vi "Automatic Teller Machine (ATM).vi"() -> ()   [LabVIEW 2019]
uses:
  Controls/UI Data.ctl
  Controls/Message selector.ctl
  SubVIs/FGV Selector.ctl
  SubVIs/Operation.ctl
  Controls/Write Menu.ctl
  support/Message Queue/Enqueue Message (Single).vi
  <vilib>/Utility/file.llb/Read Delimited Spreadsheet (string).vi
  <vilib>/Utility/file.llb/Write Delimited Spreadsheet (string).vi
  <vilib>/Utility/error.llb/Error Cluster From Error Code.vi
  <vilib>/ErrorRing/Error Ring.xnode
  support/Message Queue/Message Queue.lvlib
  support/User Event - Stop/User Event - Stop.lvlib
panel:
  in  "Enter":bool
  in  "User Input":string
  in  "Right Buttons":T1
  out "Right Menu":T2
  in  "Left Buttons":T1
  out "Left Menu":T2
  in  "Card Simulator":bool
  out "ATM Messages":string
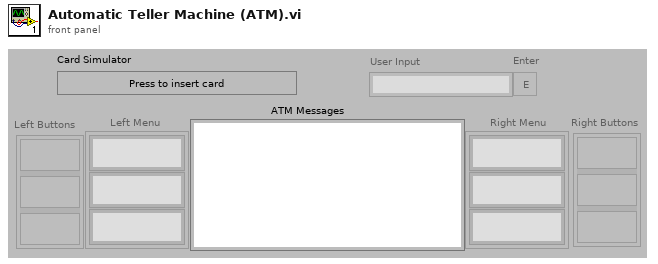
[diagram p1: front panel]
types:
  T1 = cluster{"Func Button":bool, "Func Button 2":bool, "Func Button 3":bool}
  T2 = cluster{"RFS String":string, "RFS String 2":string, "RFS String 3":string}
  T3 = typedef "UI Data.ctl" = cluster{"Account":string, "First Name":string, "Last Name":string, "Cash":i32}
  T4 = typedef "Message Queue.lvlib/All Message Queues.ctl" = cluster{"UI":refnum<queue>}
  T5 = typedef "Operation.ctl" = enum16{"No item", "Card Inserted", "Deposit", "Withdrawn"}
  T6 = typedef "FGV Selector.ctl" = enum16{"Set", "Get"}
  T7 = typedef "Message selector.ctl" = enum16{"Welcome Message", "Main Menu Message", "Account Verification Failed Message", "Session Terminate Message", "Deposit Message", "Deposit Complete Message", "Withdrawal Message", "Withdrawal Complete Message", "Withdrawal Failed Message", "Balance Inquiry Message"}
  T8 = typedef "Write Menu.ctl" = enum16{"Empty Value", "Standard Value"}
  T9 = enum8{"Enabled", "Disabled", "Disabled and Grayed Out"}
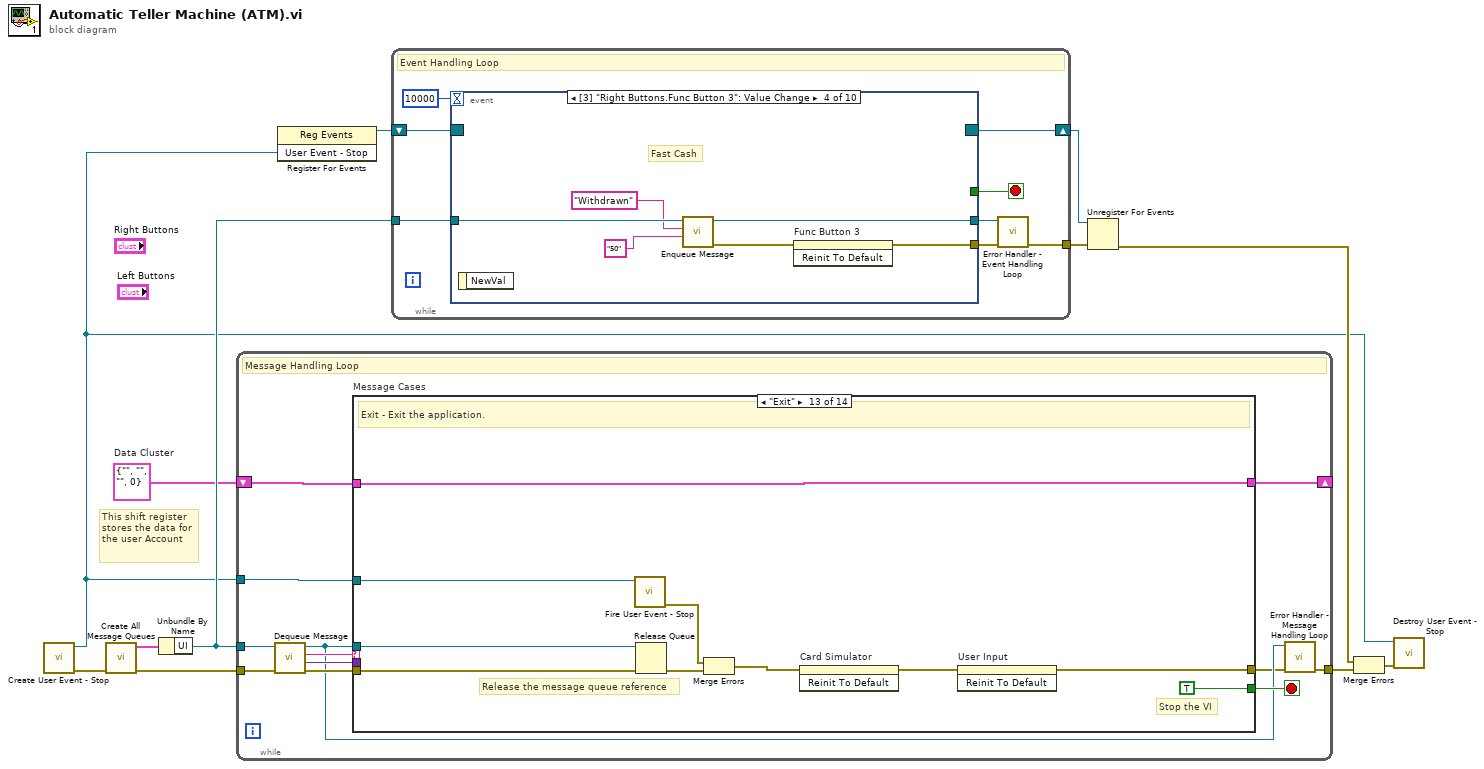
[diagram p0: block diagram]
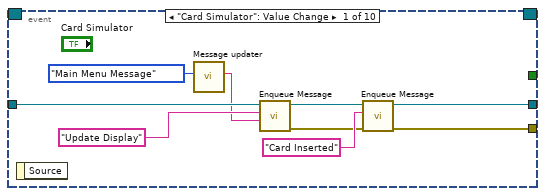
[diagram p2: hidden frame]
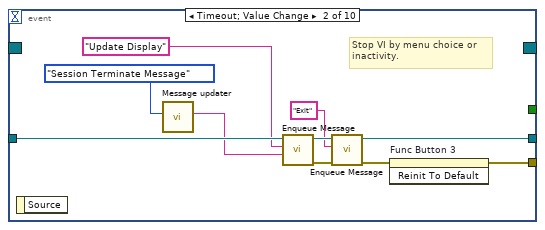
[diagram p3: hidden frame]
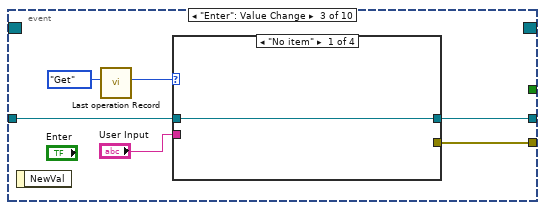
[diagram p4: hidden frame]
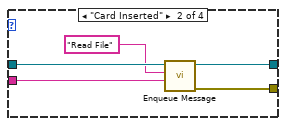
[diagram p5: hidden frame]
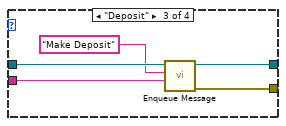
[diagram p6: hidden frame]
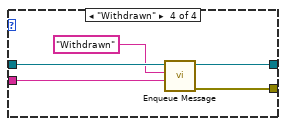
[diagram p7: hidden frame]
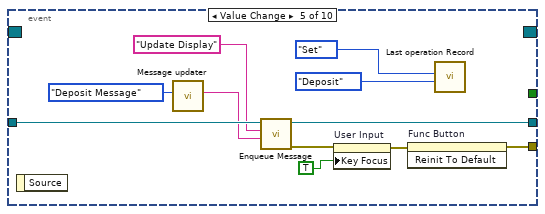
[diagram p8: hidden frame]
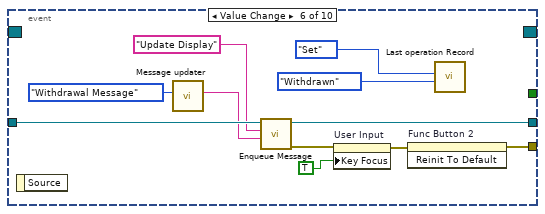
[diagram p9: hidden frame]
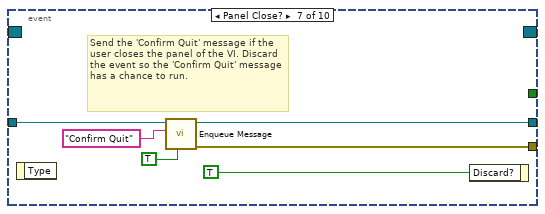
[diagram p10: hidden frame]
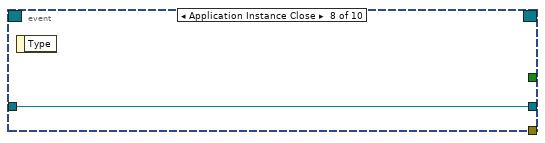
[diagram p11: hidden frame]
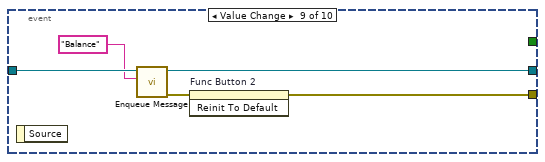
[diagram p12: hidden frame]
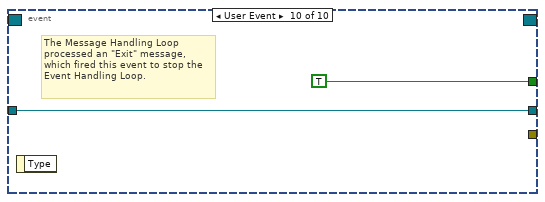
[diagram p13: hidden frame]
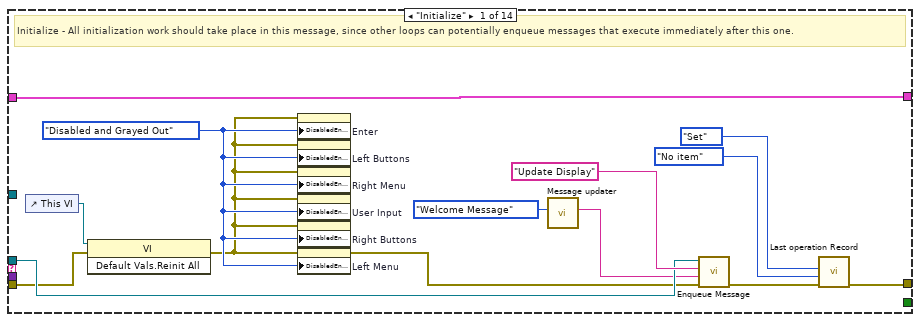
[diagram p14: hidden frame]
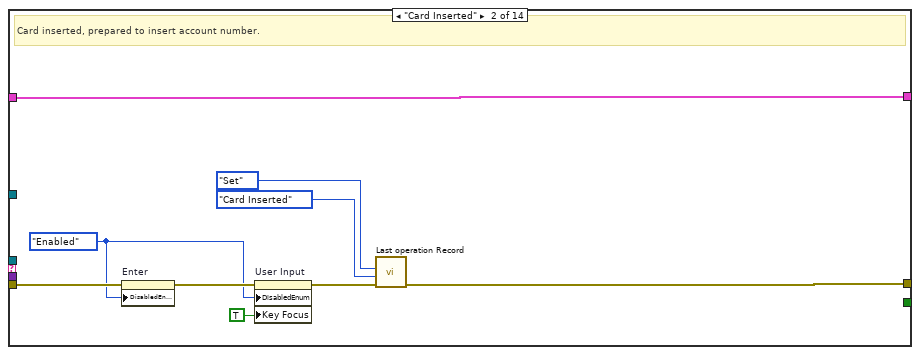
[diagram p15: hidden frame]
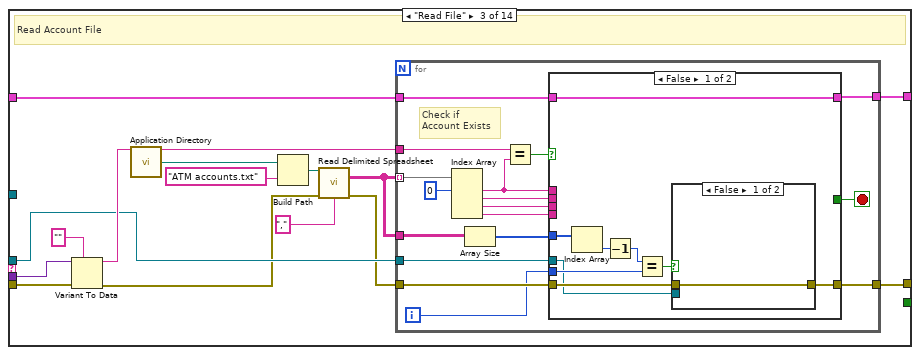
[diagram p16: hidden frame]
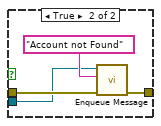
[diagram p17: hidden frame]
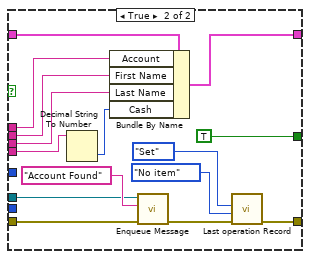
[diagram p18: hidden frame]
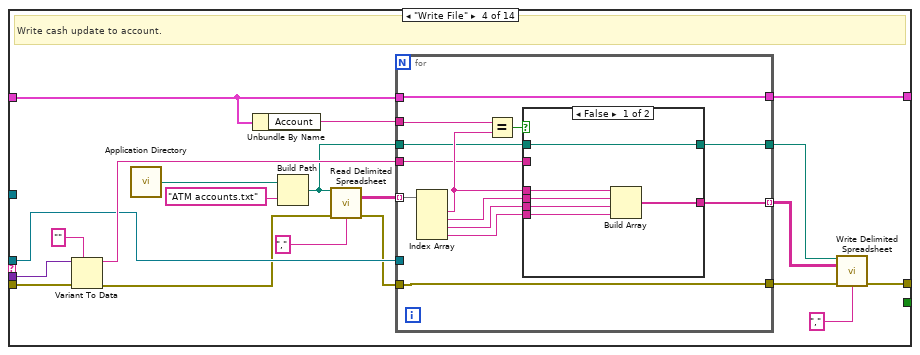
[diagram p19: hidden frame]
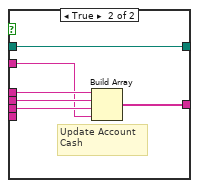
[diagram p20: hidden frame]
diagram:
  w4 = T3 {"Account"="", "First Name"="", "Last Name"="", "Cash"=0}  # Data Cluster
  # "This shift register stores the data for the user Account"
  n1 = call "Create User Event - Stop.vi"() -> ("error out"=w8:errorcluster, "User Event - Stop"=w1:refnum<user-event>)  [unwired: 10 in]
  n2 = call "Create All Message Queues.vi"("error in (no error)"=w8) -> ("error out"=w12:errorcluster, "Message Queues out"=w11:T4)  [unwired: 9 in]
  n3 = Unbundle By Name(w11) -> ("UI"=w9:refnum<queue>)
  n4 = while {
    tunnel: w9 -> [w16]
    shift-right: [w23] -> _
    shift-left: w4 -> [w24]
    tunnel: w1 -> [w21]
    tunnel: w12 -> [w20]
    tunnel: [w14] -> w10
    stop <- w22 stop-if-true
    # "Message Handling Loop"
    n5 = call "Dequeue Message.vi"("error in (no error)"=w20, "Message Queue"=w16) -> ("error out"=w19:errorcluster, "Message Data"=w17:variant, "Message"=w18:string, "dup Message Queue"=w15:refnum<queue>)  [unwired: 6 in]
    n6 = case "Message Cases" shown="\"Exit\"" w18 {
      selector: w18 -> [_ _ _ _ _ _ _ _ _ _ _ _ _ w292]
      tunnel: w15 -> [w36 _ w51 w121 w170 w183 w193 w220 w237 _ _ w278 w291 _]
      tunnel: w19 -> [w31 w45 w58 w125 w166 w181 w190 w215 w236 w268 w275 w281 w285 _]
      tunnel: [w27 w42 w53 w111 w179 w186 w197 w205 w230 w263 w270 w279 w282 w293] -> w13
      tunnel: w24 -> [w38 w47 w54 w117 w175 w184 w195 w209 w232 w269 w274 w280 w290 w294]
      tunnel: [w38 w47 w52 w114 w175 w184 w195 w207 w231 w269 w274 w280 w290 w294] -> w23
      tunnel: [_ _ _ _ _ _ _ _ _ _ _ _ TRUE _] -> w22
      tunnel: w17 -> [_ _ w57 w124 _ _ _ w214 w235 w267 w273 _ _ _]
      tunnel: w21 -> [_ _ _ _ _ _ _ _ _ _ _ _ w287 _]
      frame "Initialize" {
        w33 = T9."Disabled and Grayed Out" ("Disabled")
        # "Initialize - All initialization work should take place in this message, since other loops can potentially enqueue messages that execute immediately after this one."
        n7 = control-ref of="This VI"() -> (w32:refnum<vi>)
        n8 = invoke class="VI" method="Default Vals.Reinit All"(reference=w32, error in=w31) -> (error out=w30:errorcluster)  [unwired: 1 in, 2 out]
        n9 = property on="Enter" class="Bool"(error in=w30, "DisabledEnum"=w33) -> ()  [unwired: 1 in, 2 out]
        n10 = property on="Left Buttons" class="Clust"(error in=w30, "DisabledEnum"=w33) -> ()  [unwired: 1 in, 2 out]
        n11 = property on="Right Menu" class="Clust (strict)"(error in=w30, "DisabledEnum"=w33) -> ()  [unwired: 1 in, 2 out]
        n12 = property on="User Input" class="Str"(error in=w30, "DisabledEnum"=w33) -> ()  [unwired: 1 in, 2 out]
        n13 = property on="Right Buttons" class="Clust"(error in=w30, "DisabledEnum"=w33) -> ()  [unwired: 1 in, 2 out]
        n14 = property on="Left Menu" class="Clust (strict)"(error in=w30, "DisabledEnum"=w33) -> (error out=w29:errorcluster)  [unwired: 1 in, 1 out]
        n15 = call "Message updater.vi"("Message Selector"=Message_selector."Welcome Message") -> ("Message"=w34:string)  [unwired: 10 in]
        n16 = call-poly "Enqueue Message.vi"("error in (no error)"=w29, "Message Data"=w34, "Message"="Update Display", "Message Queue"=w36) -> ("error out"=w28:errorcluster)  [unwired: 6 in, 1 out]
        n17 = call "Last operation Record.vi"("Error In"=w28, "Operation"=Operation."No item", "FGV Choice"=FGV_Selector."Set") -> ("Error Out"=w27:errorcluster)  [unwired: 7 in, 1 out]
      }
      frame "Card Inserted" {
        w44 = T9."Enabled" ("Disabled")
        # "Card inserted, prepared to insert account number."
        n18 = property on="Enter" class="Bool"(error in=w45, "DisabledEnum"=w44) -> (error out=w46:errorcluster)  [unwired: 1 in, 1 out]
        n19 = property on="User Input" class="Str"(error in=w46, "DisabledEnum"=w44, "Key Focus"=TRUE) -> (error out=w43:errorcluster)  [unwired: 1 in, 1 out]
        n20 = call "Last operation Record.vi"("Error In"=w43, "Operation"=Operation."Card Inserted", "FGV Choice"=FGV_Selector."Set") -> ("Error Out"=w42:errorcluster)  [unwired: 7 in, 1 out]
      }
      frame "Read File" {
        # "Read Account File"
        n21 = Variant To Data(error in=w58, type="", Variant=w57) -> (data=w55:string, error out=w50:errorcluster)
        n22 = call <vilib>:"Application Directory.vi"() -> ("Application Directory"=w61:path)
        n23 = Build Path(base path=w61, name or relative path="ATM accounts.txt") -> (appended path=w59:path)
        n24 = call-poly <vilib>:"Read Delimited Spreadsheet.vi"("file path (dialog if empty)"=w59, "error in (no error)"=w50, "delimiter (\\t)"="," ("delimiter (\\t)")) -> ("all rows"=w48:string[][], "error out"=w49:errorcluster)  [unwired: 7 in, 4 out]
        n25 = for {
          tunnel: w48 -> [w79] mode=indexing
          tunnel: w49 -> [w68]
          tunnel: w55 -> [w77]
          tunnel: w54 -> [w75]
          tunnel: [w72] -> w52
          tunnel: [w70] -> w53
          tunnel: w51 -> [w69]
          tunnel: w48 -> [w67]
          i -> [w63]
          stop <- w71 stop-if-true
          # "Check if\nAccount Exists"
          n26 = Index Array(array=w79, index #1=0 ("index")) -> (element #1=w73:string, element #2=w74:string, element #3=w64:string, element #4=w65:string)  [unwired: 3 in]
          n27 = Array Size(array=w67) -> (size(s)=w66:i32[])
          n28 = Equal?(x=w77, y=w73) -> (x = y?=w76:bool)
          n29 = case shown="False" w76 {
            tunnel: w75 -> [w88 w108]
            tunnel: w74 -> [_ w106]
            tunnel: w65 -> [_ w107]
            tunnel: w73 -> [_ w105]
            tunnel: [w88 w104] -> w72
            tunnel: [_ TRUE] -> w71
            tunnel: [w80 w96] -> w70
            tunnel: w69 -> [w81 w101]
            tunnel: w68 -> [w82 w100]
            tunnel: w66 -> [w86 _]
            tunnel: w64 -> [_ w94]
            tunnel: w63 -> [w83 _]
            frame False {
              n30 = Index Array(array=w86) -> (element=w87:i32)  [unwired: 1 in]
              n31 = Decrement(x=w87) -> (x-1=w84:i32)
              n32 = Equal?(x=w84, y=w83) -> (x = y?=w85:bool)
              n33 = case shown="False" w85 {
                tunnel: w82 -> [w89 w92]
                tunnel: w81 -> [_ w91]
                tunnel: [w89 w90] -> w80
                frame False {
                }
                frame True {
                  n34 = call-poly "Enqueue Message.vi"("error in (no error)"=w92, "Message"="Account not Found", "Message Queue"=w91) -> ("error out"=w90:errorcluster)  [unwired: 7 in, 1 out]
                }
              }
            }
            frame True {
              n35 = Decimal String To Number(string=w107) -> (number=w95:i32)  [unwired: 2 in, 1 out]
              n36 = Bundle By Name(cluster=w108, "Account"=w105, "First Name"=w106, "Last Name"=w94, "Cash"=w95) -> (w104:T3)
              n37 = call-poly "Enqueue Message.vi"("error in (no error)"=w100, "Message"="Account Found", "Message Queue"=w101) -> ("error out"=w97:errorcluster)  [unwired: 7 in, 1 out]
              n38 = call "Last operation Record.vi"("Error In"=w97, "Operation"=Operation."No item", "FGV Choice"=FGV_Selector."Set") -> ("Error Out"=w96:errorcluster)  [unwired: 7 in, 1 out]
            }
          }
        }
      }
      frame "Write File" {
        # "Write cash update to account."
        n39 = Variant To Data(error in=w125, type="", Variant=w124) -> (data=w122:string, error out=w120:errorcluster)
        n40 = call <vilib>:"Application Directory.vi"() -> ("Application Directory"=w127:path)
        n41 = Unbundle By Name(w117) -> ("Account"=w116:string)
        n42 = Build Path(base path=w127, name or relative path="ATM accounts.txt") -> (appended path=w115:path)
        n43 = call-poly <vilib>:"Read Delimited Spreadsheet.vi"("file path (dialog if empty)"=w115, "error in (no error)"=w120, "delimiter (\\t)"="," ("delimiter (\\t)")) -> ("all rows"=w118:string[][], "error out"=w119:errorcluster)  [unwired: 7 in, 4 out]
        n44 = for {
          tunnel: w118 -> [w141] mode=indexing
          tunnel: w119 -> [w129]
          tunnel: w122 -> [w133]
          tunnel: w117 -> [w132]
          tunnel: w121 -> [_]
          tunnel: w116 -> [w140]
          tunnel: [w134] -> w112 mode=indexing
          tunnel: w115 -> [w131]
          tunnel: [w132] -> w114
          tunnel: [w130] -> w113
          tunnel: [w129] -> w110
          n45 = Index Array(array=w141) -> (element #1=w138:string, element #2=w137:string, element #3=w136:string, element #4=w135:string)  [unwired: 4 in]
          n46 = Equal?(x=w140, y=w138) -> (x = y?=w139:bool)
          n47 = case shown="False" w139 {
            tunnel: w138 -> [w147 w153]
            tunnel: w137 -> [w146 w152]
            tunnel: w136 -> [w145 w151]
            tunnel: w135 -> [w144 _]
            tunnel: [w143 w150] -> w134
            tunnel: w133 -> [_ w149]
            tunnel: w131 -> [w142 w148]
            tunnel: [w142 w148] -> w130
            frame False {
              n48 = Build Array(w147, w146, w145, w144) -> (w143:string[])
            }
            frame True {
              # "Update Account\nCash"
              n49 = Build Array(w153, w152, w151, w149) -> (w150:string[])
            }
          }
        }
        n50 = call-poly <vilib>:"Write Delimited Spreadsheet.vi"("file path (dialog if empty)"=w113, "2D data"=w112, "error in (no error)"=w110, "delimiter (\\t)"="," ("delimiter (\\t)")) -> ("error out"=w111:errorcluster)  [unwired: 10 in, 1 out]
      }
      frame "Account Found" {
        w167 = T9."Enabled" ("Disabled")
        # "If account was found, enable controls, menus and show message displaying customer name."
        n51 = property on="Left Buttons" class="Clust"(error in=w166, "DisabledEnum"=w167) -> (error out=w163:errorcluster)  [unwired: 1 in, 1 out]
        n52 = property on="Right Menu" class="Clust (strict)"(error in=w166, "DisabledEnum"=w167) -> (error out=w162:errorcluster)  [unwired: 1 in, 1 out]
        n53 = property on="Right Buttons" class="Clust"(error in=w166, "DisabledEnum"=w167) -> (error out=w161:errorcluster)  [unwired: 1 in, 1 out]
        n54 = property on="Left Menu" class="Clust (strict)"(error in=w166, "DisabledEnum"=w167) -> (error out=w160:errorcluster)  [unwired: 1 in, 1 out]
        n55 = Merge Errors(w163, w162, w161, w160) -> (w164:errorcluster)
        n56 = call "Write Menu Value.vi"("Error In"=w164, "Menu Write choice"=Write_Menu."Standard Value") -> ("Error Out"=w157:errorcluster, "Right Menu"=→"Right Menu":T2, "Left Menu"=→"Left Menu":T2)  [unwired: 7 in]
        n57 = call "Last operation Record.vi"("Error In"=w157, "Operation"=Operation."No item", "FGV Choice"=FGV_Selector."Set") -> ("Error Out"=w156:errorcluster)  [unwired: 7 in, 1 out]
        n58 = Unbundle By Name(w175) -> ("Last Name"=w171:string, "First Name"=w173:string)
        n59 = call "Message updater.vi"("Message Selector"=Message_selector."Main Menu Message") -> ("Message"=w177:string)  [unwired: 10 in]
        n60 = Search and Replace String(input string=w177, search string="First Name", replace string=w173) -> (result string=w176:string)  [unwired: 5 in, 3 out]
        n61 = Search and Replace String(input string=w176, search string="Last Name (from file)", replace string=w171) -> (result string=w168:string)  [unwired: 5 in, 3 out]
        n62 = call-poly "Enqueue Message.vi"("error in (no error)"=w156, "Message Data"=w168, "Message"="Update Display", "Message Queue"=w170) -> ("error out"=w179:errorcluster)  [unwired: 6 in, 1 out]
      }
      frame "Account not Found" {
        # "Send message to Display showing that account does not exist."
        n63 = call "Message updater.vi"("Message Selector"=Message_selector."Account Verification Failed Message") -> ("Message"=w180:string)  [unwired: 10 in]
        n64 = call-poly "Enqueue Message.vi"("error in (no error)"=w181, "Message Data"=w180, "Message"="Update Display", "Message Queue"=w183) -> ("error out"=w186:errorcluster)  [unwired: 6 in, 1 out]
      }
      frame "Balance" {
        # "Get Balance From account."
        n65 = Unbundle By Name(w195) -> ("Cash"=w188:i32)
        n66 = call "Message updater.vi"("Message Selector"=Message_selector."Balance Inquiry Message") -> ("Message"=w189:string)  [unwired: 10 in]
        n67 = Number To Decimal String(number=w188) -> (decimal integer string=w187:string)  [unwired: 1 in]
        n68 = Search and Replace String(input string=w189, search string="(Balance Amount from file)", replace string=w187) -> (result string=w191:string)  [unwired: 5 in, 3 out]
        n69 = call-poly "Enqueue Message.vi"("error in (no error)"=w190, "Message Data"=w191, "Message"="Update Display", "Message Queue"=w193) -> ("error out"=w197:errorcluster)  [unwired: 6 in, 1 out]
      }
      frame "Make Deposit" {
        # "Make Deposit"
        n70 = Unbundle By Name(w209) -> ("Cash"=w211:i32)
        n71 = Variant To Data(error in=w215, type="", Variant=w214) -> (data=w212:string, error out=w199:errorcluster)
        n72 = Decimal String To Number(string=w212) -> (number=w210:i32)  [unwired: 2 in, 1 out]
        n73 = Add(x=w211, y=w210) -> (x+y=w208:i32)
        n74 = Bundle By Name(cluster=w209, "Cash"=w208) -> (w207:T3)
        n75 = call "Last operation Record.vi"("Error In"=w199, "Operation"=Operation."No item", "FGV Choice"=FGV_Selector."Set") -> ("Error Out"=w198:errorcluster)  [unwired: 7 in, 1 out]
        n76 = Unbundle By Name(w207) -> ("Cash"=w216:i32)
        n77 = Number To Decimal String(number=w216) -> (decimal integer string=w202:string)  [unwired: 1 in]
        n78 = call "Message updater.vi"("Message Selector"=Message_selector."Deposit Complete Message") -> ("Message"=w217:string)  [unwired: 10 in]
        n79 = Search and Replace String(input string=w217, search string="(Amount)", replace string=w212) -> (result string=w218:string)  [unwired: 5 in, 3 out]
        n80 = call-poly "Enqueue Message.vi"("error in (no error)"=w198, "Message Data"=w218, "Message"="Update Display", "Message Queue"=w220) -> ("error out"=w204:errorcluster, "dup Message Queue"=w206:refnum<queue>)  [unwired: 6 in]
        n81 = call-poly "Enqueue Message.vi"("error in (no error)"=w204, "Message Data"=w202, "Message"="Write File", "Message Queue"=w206) -> ("error out"=w205:errorcluster)  [unwired: 6 in, 1 out]
      }
      frame "Withdrawn" {
        # "Make Deposit"
        n82 = Variant To Data(error in=w236, type="", Variant=w235) -> (data=w233:string, error out=w224:errorcluster)
        n83 = Unbundle By Name(w232) -> ("Cash"=w228:i32)
        n84 = Decimal String To Number(string=w233) -> (number=w227:i32)  [unwired: 2 in, 1 out]
        n85 = Greater Or Equal?(x=w228, y=w227) -> (x >= y?=w229:bool)
        n86 = call "Last operation Record.vi"("Error In"=w224, "Operation"=Operation."No item", "FGV Choice"=FGV_Selector."Set") -> ("Error Out"=w223:errorcluster)  [unwired: 7 in, 1 out]
        n87 = case shown="True" w229 {
          tunnel: w237 -> [w253 w261]
          tunnel: w223 -> [w249 w258]
          tunnel: w233 -> [w248 _]
          tunnel: w232 -> [w247 w257]
          tunnel: [w246 w257] -> w231
          tunnel: [w244 w256] -> w230
          tunnel: w228 -> [w240 _]
          tunnel: w227 -> [w239 _]
          frame True {
            n88 = Subtract(x=w240, y=w239) -> (x-y=w238:i32)
            n89 = Bundle By Name(cluster=w247, "Cash"=w238) -> (w246:T3)
            n90 = Number To Decimal String(number=w238) -> (decimal integer string=w241:string)  [unwired: 1 in]
            n91 = call "Message updater.vi"("Message Selector"=Message_selector."Withdrawal Complete Message") -> ("Message"=w250:string)  [unwired: 10 in]
            n92 = Search and Replace String(input string=w250, search string="(Amount)", replace string=w248) -> (result string=w251:string)  [unwired: 5 in, 3 out]
            n93 = call-poly "Enqueue Message.vi"("error in (no error)"=w249, "Message Data"=w251, "Message"="Update Display", "Message Queue"=w253) -> ("error out"=w243:errorcluster, "dup Message Queue"=w245:refnum<queue>)  [unwired: 6 in]
            n94 = call-poly "Enqueue Message.vi"("error in (no error)"=w243, "Message Data"=w241, "Message"="Write File", "Message Queue"=w245) -> ("error out"=w244:errorcluster)  [unwired: 6 in, 1 out]
          }
          frame False {
            n95 = call "Message updater.vi"("Message Selector"=Message_selector."Withdrawal Failed Message") -> ("Message"=w259:string)  [unwired: 10 in]
            n96 = call-poly "Enqueue Message.vi"("error in (no error)"=w258, "Message Data"=w259, "Message"="Update Display", "Message Queue"=w261) -> ("error out"=w256:errorcluster)  [unwired: 6 in, 1 out]
          }
        }
      }
      frame "Update Display" {
        # "Update Display - Convert the message data to a string to display in the Data Display indicator."
        n97 = Variant To Data(error in=w268, type="", Variant=w267) -> (data=→"ATM Messages":string, error out=w264:errorcluster)
        n98 = invoke on="User Input" class="Str" method="Reinit To Default"(error in=w264) -> (error out=w263:errorcluster)  [unwired: 2 in, 2 out]
      }
      frame "Error" {
        # "Error - Display an error dialog. This message is sent by the \"Error Handler\" VIs at the end of other loops in this application."
        n99 = Variant To Data(error in=w275, type=errorcluster {"status"=FALSE, "code"=0, "source"=""} ("error constant"), Variant=w273) -> (data=w271:errorcluster, error out=w270:errorcluster)
        n100 = call <vilib>:"Simple Error Handler.vi"("error in (no error)"=w271) -> ()  [unwired: 4 in, 5 out]
      }
      frame "Confirm Quit" {
        # "Confirm Quit - Message that can confirm whether or not the user wants to exit the application."
        n101 = call-poly "Enqueue Message.vi"("Priority Message? (F)"=TRUE, "error in (no error)"=w281, "Message"="Exit", "Message Queue"=w278) -> ("error out"=w279:errorcluster)  [unwired: 6 in, 1 out]
      }
      frame "Exit" {
        # "Stop the VI"
        # "Release the message queue reference"
        # "Exit - Exit the application."
        n102 = call "Fire User Event - Stop.vi"("User Event - Stop"=w287) -> ("error out"=w286:errorcluster)  [unwired: 10 in]
        n103 = Release Queue(queue=w291, error in (no error)=w285) -> (error out=w288:errorcluster)  [unwired: 1 in, 2 out]
        n104 = Merge Errors(w286, w288) -> (w284:errorcluster)
        n105 = invoke on="Card Simulator" class="Bool (strict)" method="Reinit To Default"(error in=w284) -> (error out=w283:errorcluster)  [unwired: 2 in, 2 out]
        n106 = invoke on="User Input" class="Str" method="Reinit To Default"(error in=w283) -> (error out=w282:errorcluster)  [unwired: 2 in, 2 out]
      }
      frame Default {
        # "'Default' case only runs if there is a message that isn't defined in any of the other cases.  Output a programming error."
        n107 = xnode "Error Ring"("parameter 0"=w292) -> ("error out"=w293:errorcluster)
      }
    }
    n108 = call "Error Handler - Message Handling Loop.vi"("error in (no error)"=w13, "Message Queue"=w15) -> ("dup error in"=w14:errorcluster)  [unwired: 8 in, 1 out]
  }
  n109 = register-events(w1) -> (reference out=w2:refnum<event-registration>)  [unwired: 2 in, 1 out]
  n110 = while {
    tunnel: w9 -> [w309]
    shift-right: [w307] -> w5
    shift-left: w2 -> [w308]
    tunnel: [w303] -> w3
    stop <- w305 stop-if-true
    # "Event Handling Loop"
    n111 = event shown="[3] \"Right Buttons.Func Button 3\": Value Change" {
      selector: w308 -> [_ _ _ _ _ _ _ _ _ _]
      dyn-events: [_ _ _ _ _ _ _ _ _ _] -> w307
      timeout: 10000 -> [_ _ _ _ _ _ _ _ _ _]
      tunnel: [_ _ _ _ _ _ _ _ _ TRUE ("Discard?")] -> w305
      tunnel: w309 -> [w318 w327 w334 w356 w365 w376 w383 w385 w390 w392]
      tunnel: [w310 w319 w330 w352 w367 w378 w382 _ w386 _] -> w306
      tunnel: [w312 w322 w333 w355 w364 w375 w381 w385 w389 w392] -> w304
      event "Card Simulator": Value Change {
        n112 = event-data() -> ()  [unwired: 1 in, 1 out]
        n113 = call "Message updater.vi"("Message Selector"=Message_selector."Main Menu Message") -> ("Message"=w316:string)  [unwired: 10 in]
        n114 = call-poly "Enqueue Message.vi"("Message Data"=w316, "Message"="Update Display", "Message Queue"=w318) -> ("error out"=w311:errorcluster, "dup Message Queue"=w313:refnum<queue>)  [unwired: 7 in]
        n115 = call-poly "Enqueue Message.vi"("error in (no error)"=w311, "Message"="Card Inserted", "Message Queue"=w313) -> ("error out"=w310:errorcluster, "dup Message Queue"=w312:refnum<queue>)  [unwired: 7 in]
      }
      event Timeout; "Left Buttons.Func Button 3": Value Change {
        # "Stop VI by menu choice or\ninactivity."
        n116 = event-data() -> ()  [unwired: 1 in, 1 out]
        n117 = call "Message updater.vi"("Message Selector"=Message_selector."Session Terminate Message") -> ("Message"=w326:string)  [unwired: 10 in]
        n118 = call-poly "Enqueue Message.vi"("Message Data"=w326, "Message"="Update Display", "Message Queue"=w327) -> ("error out"=w323:errorcluster, "dup Message Queue"=w324:refnum<queue>)  [unwired: 7 in]
        n119 = call-poly "Enqueue Message.vi"("error in (no error)"=w323, "Message"="Exit", "Message Queue"=w324) -> ("error out"=w320:errorcluster, "dup Message Queue"=w322:refnum<queue>)  [unwired: 7 in]
        n120 = invoke on="Func Button 3" class="Bool" method="Reinit To Default"(error in=w320) -> (error out=w319:errorcluster)  [unwired: 2 in, 2 out]
      }
      event "Enter": Value Change {
        n121 = event-data() -> ()  [unwired: 1 in, 1 out]
        n122 = call "Last operation Record.vi"("FGV Choice"=FGV_Selector."Get") -> ("Last Operation"=w332:T5)  [unwired: 9 in, 1 out]
        n123 = case shown="\"No item\"" w332 {
          tunnel: w334 -> [w335 w338 w343 w348]
          tunnel: [w335 w339 w344 w349] -> w333
          tunnel: [_ w340 w345 w350] -> w330
          tunnel: "User Input" -> [_ w336 w341 w346]
          frame "No item" {
          }
          frame "Card Inserted" {
            n124 = call-poly "Enqueue Message.vi"("Message Data"=w336, "Message"="Read File", "Message Queue"=w338) -> ("error out"=w340:errorcluster, "dup Message Queue"=w339:refnum<queue>)  [unwired: 7 in]
          }
          frame "Deposit" {
            n125 = call-poly "Enqueue Message.vi"("Message Data"=w341, "Message"="Make Deposit", "Message Queue"=w343) -> ("error out"=w345:errorcluster, "dup Message Queue"=w344:refnum<queue>)  [unwired: 7 in]
          }
          frame "Withdrawn" {
            n126 = call-poly "Enqueue Message.vi"("Message Data"=w346, "Message"="Withdrawn", "Message Queue"=w348) -> ("error out"=w350:errorcluster, "dup Message Queue"=w349:refnum<queue>)  [unwired: 7 in]
          }
        }
      }
      event "Right Buttons.Func Button 3": Value Change {
        # "Fast Cash"
        n127 = event-data() -> ()  [unwired: 1 in, 1 out]
        n128 = call-poly "Enqueue Message.vi"("Message Data"="50", "Message"="Withdrawn", "Message Queue"=w356) -> ("error out"=w351:errorcluster, "dup Message Queue"=w355:refnum<queue>)  [unwired: 7 in]
        n129 = invoke on="Func Button 3" class="Bool" method="Reinit To Default"(error in=w351) -> (error out=w352:errorcluster)  [unwired: 2 in, 2 out]
      }
      event "Right Buttons.Func Button": Value Change {
        n130 = event-data() -> ()  [unwired: 1 in, 1 out]
        n131 = call "Message updater.vi"("Message Selector"=Message_selector."Deposit Message") -> ("Message"=w363:string)  [unwired: 10 in]
        n132 = call-poly "Enqueue Message.vi"("Message Data"=w363, "Message"="Update Display", "Message Queue"=w365) -> ("error out"=w361:errorcluster, "dup Message Queue"=w364:refnum<queue>)  [unwired: 7 in]
        n133 = property on="User Input" class="Str"(error in=w361, "Key Focus"=TRUE) -> (error out=w360:errorcluster)  [unwired: 1 in, 1 out]
        n134 = invoke on="Func Button" class="Bool" method="Reinit To Default"(error in=w360) -> (error out=w367:errorcluster)  [unwired: 2 in, 2 out]
        n135 = call "Last operation Record.vi"("Operation"=Operation."Deposit", "FGV Choice"=FGV_Selector."Set") -> ()  [unwired: 8 in, 2 out]
      }
      event "Right Buttons.Func Button 2": Value Change {
        n136 = event-data() -> ()  [unwired: 1 in, 1 out]
        n137 = call "Message updater.vi"("Message Selector"=Message_selector."Withdrawal Message") -> ("Message"=w374:string)  [unwired: 10 in]
        n138 = call-poly "Enqueue Message.vi"("Message Data"=w374, "Message"="Update Display", "Message Queue"=w376) -> ("error out"=w372:errorcluster, "dup Message Queue"=w375:refnum<queue>)  [unwired: 7 in]
        n139 = property on="User Input" class="Str"(error in=w372, "Key Focus"=TRUE) -> (error out=w371:errorcluster)  [unwired: 1 in, 1 out]
        n140 = invoke on="Func Button 2" class="Bool" method="Reinit To Default"(error in=w371) -> (error out=w378:errorcluster)  [unwired: 2 in, 2 out]
        n141 = call "Last operation Record.vi"("Operation"=Operation."Withdrawn", "FGV Choice"=FGV_Selector."Set") -> ()  [unwired: 8 in, 2 out]
      }
      event Panel Close? {
        # "Send the 'Confirm Quit' message if the user closes the panel of the VI. Discard the event so the 'Confirm Quit' message has a chance to run."
        n142 = event-data() -> ()  [unwired: 1 in, 1 out]
        n143 = call-poly "Enqueue Message.vi"("Priority Message? (F)"=TRUE, "Message"="Confirm Quit", "Message Queue"=w383) -> ("error out"=w382:errorcluster, "dup Message Queue"=w381:refnum<queue>)  [unwired: 7 in]
        n144 = event-data("Discard?"=TRUE) -> ()  [unwired: 1 in, 1 out]
      }
      event Application Instance Close {
        n145 = event-data() -> ()  [unwired: 1 in, 1 out]
      }
      event "Left Buttons.Func Button 2": Value Change {
        n146 = event-data() -> ()  [unwired: 1 in, 1 out]
        n147 = call-poly "Enqueue Message.vi"("Message"="Balance", "Message Queue"=w390) -> ("error out"=w387:errorcluster, "dup Message Queue"=w389:refnum<queue>)  [unwired: 8 in]
        n148 = invoke on="Func Button 2" class="Bool" method="Reinit To Default"(error in=w387) -> (error out=w386:errorcluster)  [unwired: 2 in, 2 out]
      }
      event User Event {
        # "The Message Handling Loop processed an \"Exit\" message, which fired this event to stop the Event Handling Loop."
        n149 = event-data() -> ()  [unwired: 1 in, 1 out]
      }
    }
    n150 = call "Error Handler - Event Handling Loop.vi"("error in (no error)"=w306, "Message Queue"=w304) -> ("dup error in"=w303:errorcluster)  [unwired: 8 in, 1 out]
  }
  n151 = Unregister For Events(event registration refnum=w5, error in=w3) -> (error out=w6:errorcluster)
  n152 = Merge Errors(w6, w10) -> (w7:errorcluster)
  n153 = call "Destroy User Event - Stop.vi"("error in (no error)"=w7, "User Event - Stop"=w1) -> ()  [unwired: 9 in, 1 out]
